vi "Liste valves emballage.vi"() -> ()   [LabVIEW 2011]
panel:
  out "tableau":string[][](array[string])
  in  "chemin du fichier (utiliser une boîte de dialogue)":path=path "\\\\Plz-inf-nas\\Medic/PARAMETRES_TESTS/PROD_Data-Admin/correspondance produit code bar pour emballage.txt"
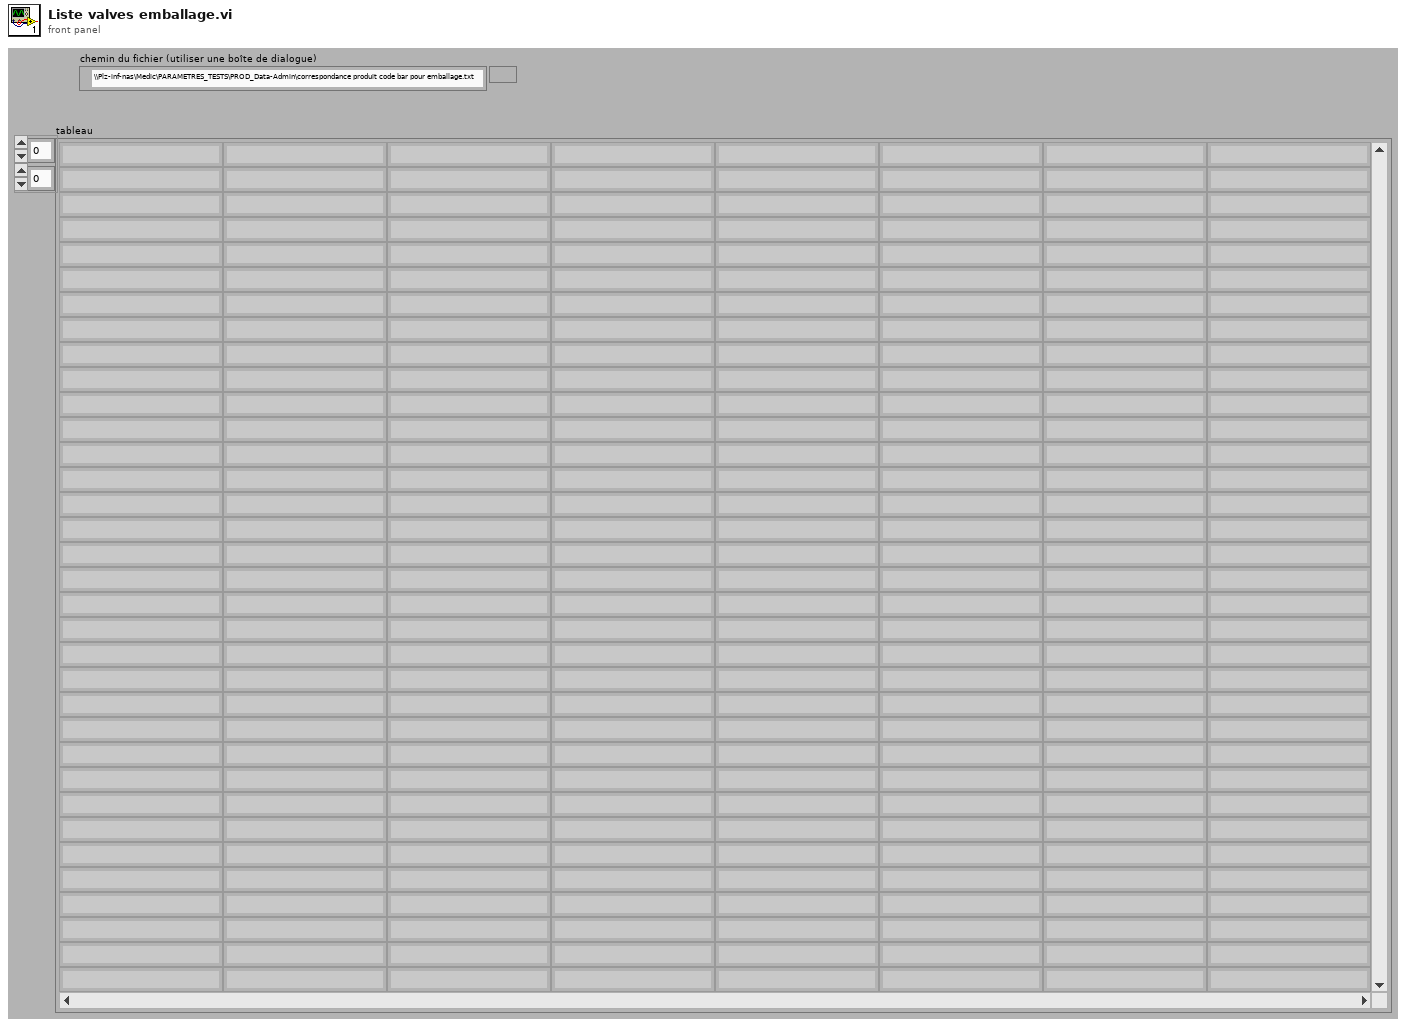
[diagram p1: front panel]
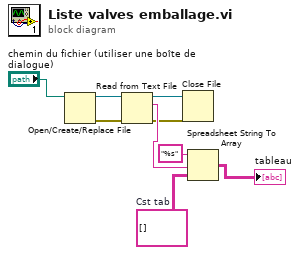
[diagram p0: block diagram]
diagram:
  w5 = string[][] []  # Cst tab
  n1 = Open/Create/Replace File(file path (use dialog)="chemin du fichier (utiliser une boîte de dialogue)") -> (refnum out=w7:refnum<file>, error out=w8:errorcluster)  [unwired: 5 in, 1 out]
  n2 = Read from Text File(file (use dialog)=w7, error in=w8) -> (refnum out=w6:refnum<file>, text=w3:string, error out=w1:errorcluster)  [unwired: 2 in, 1 out]
  n3 = Close File(refnum=w6, error in=w1) -> ()  [unwired: 2 out]
  n4 = Spreadsheet String To Array(format string="%s", spreadsheet string=w3, array type (2D Dbl)=w5) -> (array=→"tableau":string[][])  [unwired: 1 in]
